vi "Create.vi"(8 "error in (no error)":errorcluster, 9 "ID":i32, 10 "Name":string, 11 "Motor in":refnum<class "Motor.lvclass">) -> (0 "error out":errorcluster, 3 "Motor out":refnum<class "Motor.lvclass">)   [LabVIEW 2013, in "PowderDeposition.lvlib" / "Motor.lvclass"]
uses:
  Motor.lvclass
  Motor.lvclass/Motor.ctl
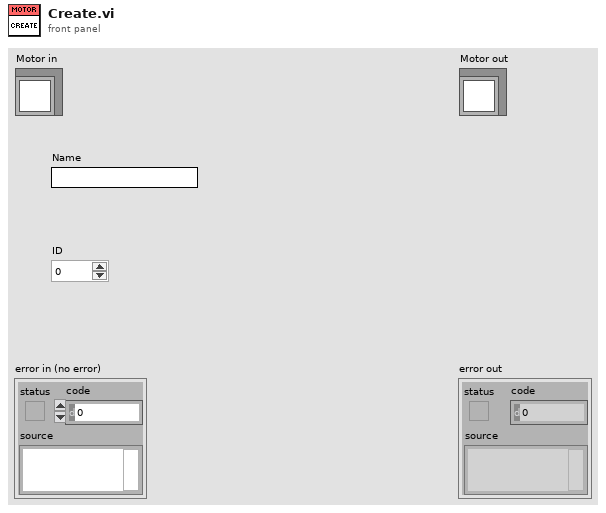
[diagram p1: front panel]
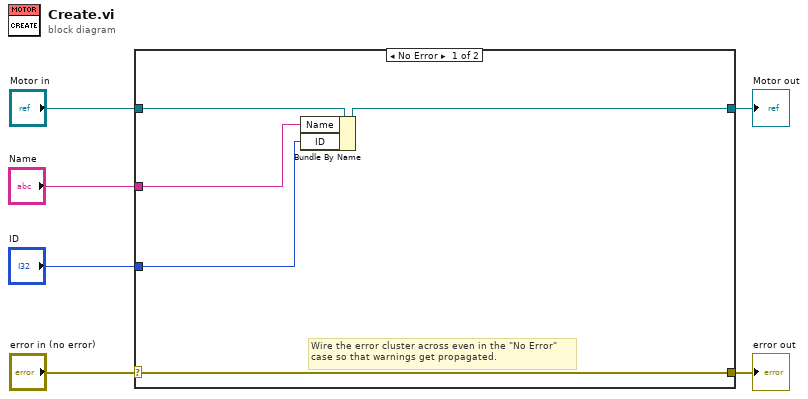
[diagram p0: block diagram]
diagram:
  n1 = case shown="No Error" "error in (no error)" {
    selector: "error in (no error)" -> [w10 w13]
    tunnel: [w10 w13] -> w5
    tunnel: [w9 w12] -> w3
    tunnel: "Motor in" -> [w11 w12]
    tunnel: "Name" -> [w8 _]
    tunnel: "ID" -> [w7 _]
    frame No Error {
      # "Wire the error cluster across even in the \"No Error\"\ncase so that warnings get propagated."
      n2 = Bundle By Name(cluster=w11, "Name"=w8, "ID"=w7) -> (w9:refnum<class "Motor.lvclass">)
    }
    frame Error {
    }
  }
  "error out" <- w5
  "Motor out" <- w3
